vi "KH_DAQ_ReadAll.vi"(8 "err in":errorcluster caption="error", 9 "Debug_DI":bool[](array[boolean]), 10 "Debug_AI":sgl[](array[numeric]), 11 "EIP_AI":T1 {"Offset" format="%.4f"; "Phys Max" format="%.4f"; "Phys Min" format="%.4f"}) -> (0 "err out":errorcluster caption="error")   [LabVIEW 2021]
uses:
  KH_DAQ_TypeDefs_Cluster AI.ctl
  KH_DAQ_TypeDefs_Messbereich.ctl
  KH EthernetIPConfig 17.14/KH EthernetIPConfig TypeDefs ModuleTyp.ctl
  KH_DAQ_TypeDefs_Bereich.ctl
  KH Turck EthernetIP 17.12/KH TURCK TypeDefs FGlob.ctl
  KH EthernetIP 17.19/KH_EthernetIP_Globals.vi
  Turck/KH_DAQ_TURCK_Global.vi
  KH Turck EthernetIP 17.12/KH TURCK ETHERNETIP Global.vi
  KH Turck EthernetIP 17.12/KH TURCK ETHERNETIP RFID Global.vi
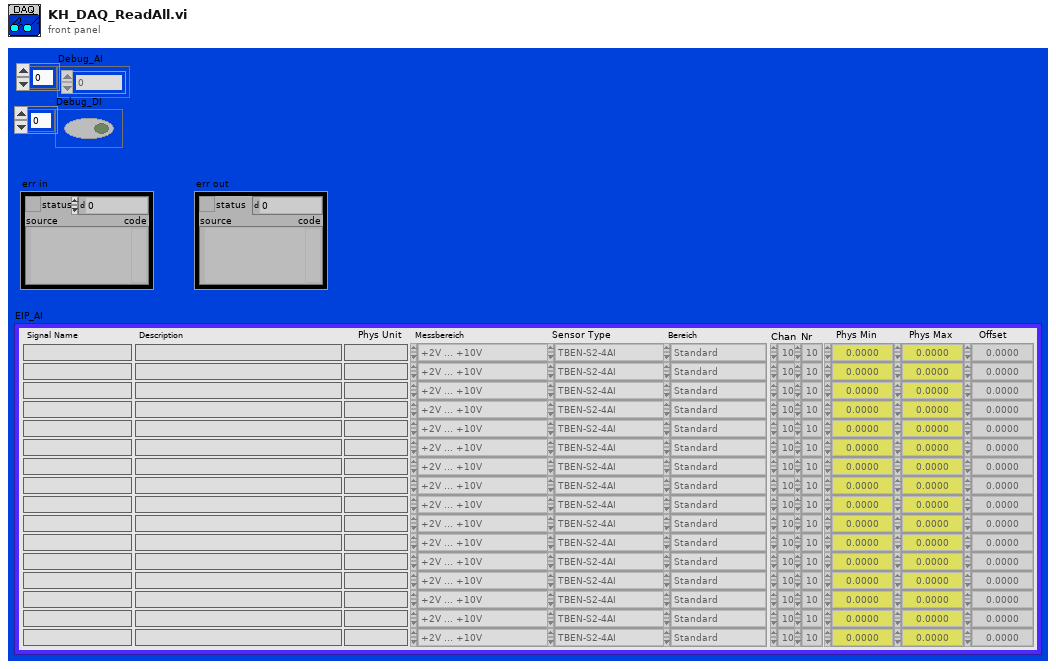
[diagram p1: front panel]
types:
  T1 = typedef "KH_DAQ_TypeDefs_Cluster AI.ctl" = cluster{"Signal Name":string[], "Description":string[], "Phys Unit":string[], "Messbereich":T2[], "Chan":u16[], "Phys Min":sgl[], "Phys Max":sgl[], "Offset":sgl[], "Nr":u16[], "SensorType 2":T3[], "Bereich":T4[]}
  T2 = typedef "KH_DAQ_TypeDefs_Messbereich.ctl" = enum16{"-10V ... +10V", "0V ... +10V", "+2V ... +10V", "0V ... +5V", "+1V ... +5V", "-1V ... +1V", "-500mV ... +500mV", "-100mV ... +100mV", "-50mV ... +50mV", "0mA ... +20mA", "+4mA ... +20mA", "-20mA ... +20mA", "0 Ohm ... 100 Ohm", "0 Ohm ... 400 Ohm", "0 Ohm ... 2000 Ohm", "0 Ohm ... 4000 Ohm", "-200°C ... 150°C PT100", "-200°C ... 150°C PT200", "-200°C ... 150°C PT500", "-200°C ... 150°C PT1000", "-60°C ... 150°C Ni100", "-60°C ... 150°C Ni1000", "-200°C ... 850°C PT100", "-200°C ... 850°C PT200", "-200°C ... 850°C PT500", "-200°C ... 850°C PT1000", "-50°C ... 250°C Ni100", "-50°C ... 250° Ni 1000"}
  T3 = typedef "KH EthernetIPConfig TypeDefs ModuleTyp.ctl" = enum16{"TBEN-S2-4AI", "TBEN-S1-8DXP", "TBEN-S2-2RFID-4DXP", "TBEN-S2-4AO", "TBEN-S2-4IOL"}
  T4 = typedef "KH_DAQ_TypeDefs_Bereich.ctl" = enum16{"Standard", "extended Range", "NE43", ""}
  T5 = typedef "KH TURCK TypeDefs FGlob.ctl" = enum16{"Put one", "Put all", "Recall one", "Recall all"}
  T6 = cluster{"ItemCount":u16, "AdressItem":cluster{"TypeID":u16, "Length":u16, "Data":cluster{"ConnectionIdentifier":u32, "SequenceNumber":u32}}, "DataItem":cluster{"TypeID":u16, "Length":u16, "Data":u8[], "Sequence Count":u16}}
  T7 = typedef "KH EthernetIPConfig TDef Config.ctl" = cluster{"Typ":T3, "Name":string, "Nr.":i32, "InputOutput":enum16{"Input", "Output"}[]}
  T8 = typedef "KH TURCK ETHERNETIP TDefCluster TBEN-S2-4AI Input Values.ctl" = cluster{"Data":i16[], "upper Limit CH0":bool, "upper Limit CH1":bool, "upper Limit CH2":bool, "upper Limit CH3":bool, "Overflow CH0":bool, "Overflow CH1":bool, "Overflow CH2":bool, "Overflow CH3":bool, "Underflow CH0":bool, "Underflow CH1":bool, "Underflow CH2":bool, "Underflow CH3":bool, "CJC Wire Break CH0":bool, "CJC Wire Break CH1":bool, "CJC Wire Break CH2":bool, "CJC Wire Break CH3":bool, "Overcurrent (RTD) CH0":bool, "Overcurrent (RTD) CH1":bool, "Overcurrent (RTD) CH2":bool, "Overcurrent (RTD) CH3":bool, "Wire Break CH0":bool, "Wire Break CH1":bool, "Wire Break CH2":bool, "Wire Break CH3":bool, "Overcurrent supply VAUX1 CH0":bool, "Overcurrent supply VAUX1 CH1":bool, "Overcurrent supply VAUX1 CH2":bool, "Overcurrent supply VAUX1 CH3":bool, "Lower limit value underrun CH0":bool, "Lower limit value underrun CH1":bool, "Lower limit value underrun CH2":bool, "Lower limit value underrun CH3":bool, "Module Diagnostics Available":bool, "INFO: ARGEE Project Running":bool, "Undervoltage Field Supply V2":bool, "Undervoltage Field Supply V1":bool, "Internal Error":bool, "Force Mode Enabled":bool}
  T9 = typedef "KH TURCK ETHERNETIP TDefCluster TBEN-S2-4AO Input Values.ctl" = cluster{"Overload Ch0":bool, "Overload Ch1":bool, "Overload Ch2":bool, "Overload Ch3":bool, "Wirebreak Ch0":bool, "Wirebreak Ch1":bool, "Wirebreak Ch2":bool, "Wirebreak Ch3":bool, "Module Diagnostics Available":bool, "INFO: ARGEE Project Running":bool, "Undervoltage V2":bool, "Undervoltage V1":bool, "Internal Error":bool, "Force Mode Enabled":bool}
  T10 = typedef "KH TURCK ETHERNETIP TDefCluster TBEN-S1-8DXP Input Values.ctl" = cluster{"Data":bool[], "Overcurrent":bool[], "Overcurrent VAUX1 Ch0-3":bool, "Overcurrent VAUX2 Ch4-7":bool, "Latch Input":bool[], "Counter value":u32, "Counter frequency (Hz)":u16, "Status":u8, "Overcurrent PWM Output 3":u8, "Overcurrent PWM Output 7":u8, "Module Diagnostics Available":bool, "INFO: ARGEE Project Running":bool, "Undervoltage V2":bool, "Undervoltage V1":bool, "Force Mode Enabled":bool}
  T11 = typedef "KH TURCK ETHERNETIP TDefCluster TBEN-S2-2RFID-4DXP Input Values.ctl" = cluster{"Station Status Word (Input Data Mapping)":cluster{"Module diagnostics avaliable":bool, "INFO: ARGEE Project Running":bool, "Undervoltage V2":bool, "Undervoltage V1":bool, "Internal Error":bool, "I/O-ASSISTANT Force Mode active":bool}, "RFID control/status 0 (Input Data Mapping)":cluster{"Tag present at r/w head":bool[], "response code":u16, "loop counter":u8, "Length":u16, "Error code":u16, "Tag counter":u16, "Data (Bytes) available":u16, "Read fragment No.":u8, "Write fragment No.":u8, "Tag present at r/w head bit":bool, "HF r/w head switched on":bool, "Continuous mode active":bool, "Antenna detuned at HF read/write head":bool, "Parameter not supported by read/write head":bool, "Error reported by read/write head":bool, "Not connected to read/write head":bool}, "RFID read data 0 (Input Data Mapping)":u8[], "RFID control/status 1 (Input Data Mapping)":cluster{"response code":u16, "Loop counter":u8, "Length":u16, "Error code":u16, "Tag counter":u16, "Data (Bytes) available":u16, "Read fragment No.":u8, "Write fragment No.":u8, "Tag present at r/w head bit":bool, "HF r/w head switched on":bool, "Continuous mode active":bool, "Antenna detuned at HF read/write head":bool, "Parameter not supported by read/write head":bool, "Error reported by read/write head":bool, "Not connected to read/write head":bool, "Tag present at r/w head":bool[]}, "RFID read data 1 (Input Data Mapping)":u8[], "RFID diagnostics (Input Data Mapping)":cluster{"Overcurrent supply VAUX1 (a)":bool, "Parameterization error (a)":bool, "Configuration via DTM active (a)":bool, "Buffer full (a)":bool, "Antenna detuned at HF read/write head (a)":bool[], "Parameter not supported by read/write head (a)":bool[], "Error reported by read/write head (a)":bool[], "Not connected to read/write head (a)":bool[], "Overcurrent supply VAUX1 (b)":bool, "Parameterization error (b)":bool, "Configuration via DTM active (b)":bool, "Buffer full (b)":bool, "Antenna detuned at HF read/write head (b)":bool[], "Parameter not supported by read/write head (b)":bool[], "Error reported by read/write head (b)":bool[], "Not connected to read/write head (b)":bool[]}, "DXP diagnostics (Input Data Mapping)":cluster{"Overcurrent VAUX2 Ch4/5":bool, "Overcurrent VAUX2 Ch6/7":bool, "Channel 4 - Output overcurrent":bool, "Channel 5 - Output overcurrent":bool, "Channel 6 - Output overcurrent":bool, "Channel 7 - Output overcurrent":bool}, "DXP (Input Data Mapping)":cluster{"Channel 4 - Input value":bool, "Channel 5 - Input value":bool, "Channel 6 - Input value":bool, "Channel 7 - Input value":bool}}
  T12 = typedef "KH TURCK ETHERNETIP TDef Enum IOL Data.ctl" = cluster{"Data_Port1":u16[], "Data_Port3":u16[], "Data_Port5":u16[], "Data_Port7":u16[], "Status":cluster{"Undervoltage Field Supply V2":bool, "Overvoltage Field Supply V1":bool, "Undervoltage Field Supply V1":bool, "Internal Error":bool, "Module Diagnostics Available":bool, "Station Configuration Changed":bool, "Overcurrent Isys":bool, "Overvoltage Field Supply V2":bool, "Force Mode Enabled":bool}, "Diagnostics":cluster{"Channel 2 - Output signal overcurrent":bool, "Channel 4 - Output signal overcurrent":bool, "Channel 6 - Output signal overcurrent":bool, "Channel 8 - Output signal overcurrent":bool, "Channel 1 - Wrong or missing device":bool, "Channel 3 - Wrong or missing device":bool, "Channel 5 - Wrong or missing device":bool, "Channel 7 - Wrong or missing device":bool, "Channel 1 - Data storage error":bool, "Channel 3 - Data storage error":bool, "Channel 5 - Data storage error":bool, "Channel 7 - Data storage error":bool, "Channel 1 - Process input data invalid":bool, "Channel 3 - Process input data invalid":bool, "Channel 5 - Process input data invalid":bool, "Channel 7 - Process input data invalid":bool, "Channel 1 - Hardware error":bool, "Channel 3 - Hardware error":bool, "Channel 5 - Hardware error":bool, "Channel 7 - Hardware error":bool, "Channel 1 - Maintenance events":bool, "Channel 3 - Maintenance events":bool, "Channel 5 - Maintenance events":bool, "Channel 7 - Maintenance events":bool, "Channel 1 - Out of spec. error":bool, "Channel 3 - Out of spec. error":bool, "Channel 5 - Out of spec. error":bool, "Channel 7 - Out of spec. error":bool, "Channel 1 - Parameterization error":bool, "Channel 3 - Parameterization error":bool, "Channel 5 - Parameterization error":bool, "Channel 1 - Overtemperature":bool, "Channel 3 - Overtemperature":bool, "Channel 5 - Overtemperature":bool, "Channel 7 - Overtemperature":bool, "Channel 1 - Lower limit value underrun":bool, "Channel 3 - Lower limit value underrun":bool, "Channel 5 - Lower limit value underrun":bool, "Channel 7 - Lower limit value underrun":bool, "Channel 1 - Upper limit value exceeded":bool, "Channel 3 - Upper limit value exceeded":bool, "Channel 5 - Upper limit value exceeded":bool, "Channel 7 - Upper limit value exceeded":bool, "Channel 1 - Undervoltage":bool, "Channel 3 - Undervoltage":bool, "Channel 5 - Undervoltage":bool, "Channel 7 - Undervoltage":bool, "Channel 1 - Overvoltage":bool, "Channel 3 - Overvoltage":bool, "Channel 5 - Overvoltage":bool, "Channel 7 - Overvoltage":bool, "Channel 1 - Overload":bool, "Channel 3 - Overload":bool, "Channel 5 - Overload":bool, "Channel 7 - Overload":bool, "Channel 1 - Common error":bool, "Channel 3 - Common error":bool, "Channel 5 - Common error":bool, "Channel 7 - Common error":bool, "Channel 1 - Port parameterization error":bool, "Channel 3 - Port parameterization error":bool, "Channel 5 - Port parameterization error":bool, "Channel 7 - Parameterization error":bool, "Channel 7 - Port parameterization error":bool}, "Events":cluster{"Event":u8[], "Qualifier":u8[], " Event code":u16[]}, "DXP":cluster{"DI Input value 2":bool, "DI Input value 4":bool, "DI Input value 6":bool, "DI Input value 8":bool, "DI Input 1":bool, "DI Input 3":bool, "DI Input 5":bool, "DI Input 7":bool, "Input values valid 1":bool, "Input values valid 3":bool, "Input values valid 5":bool, "Input values valid 7":bool}}
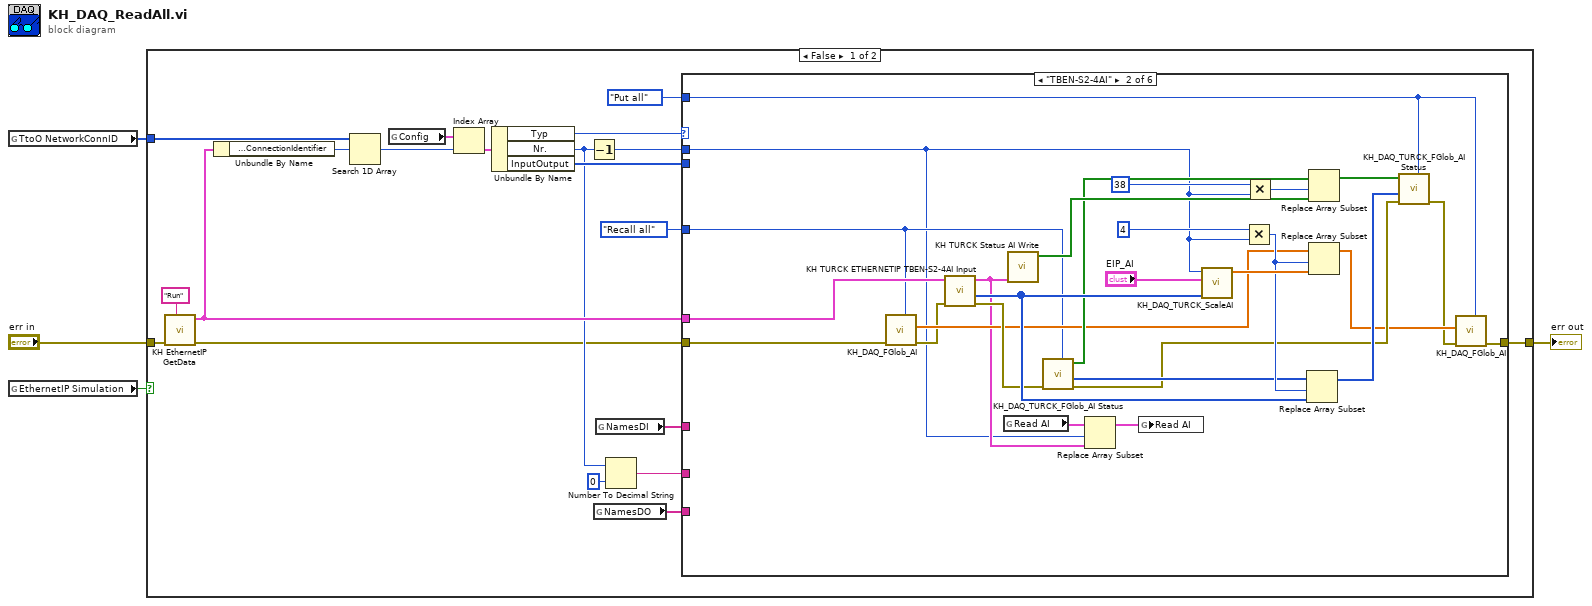
[diagram p0: block diagram]
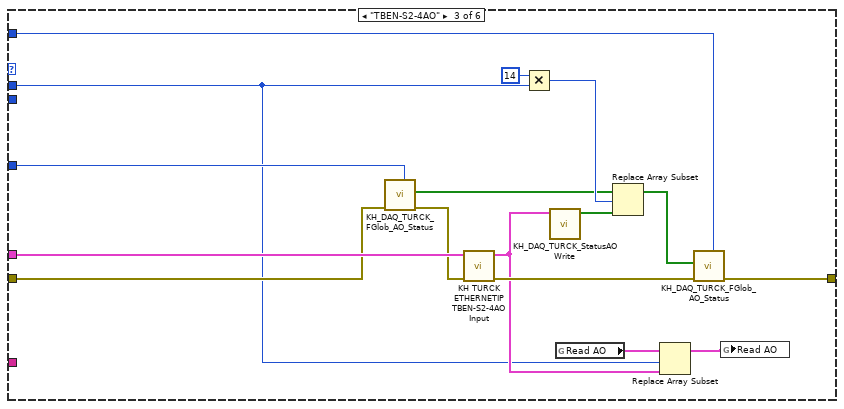
[diagram p3: hidden frame]
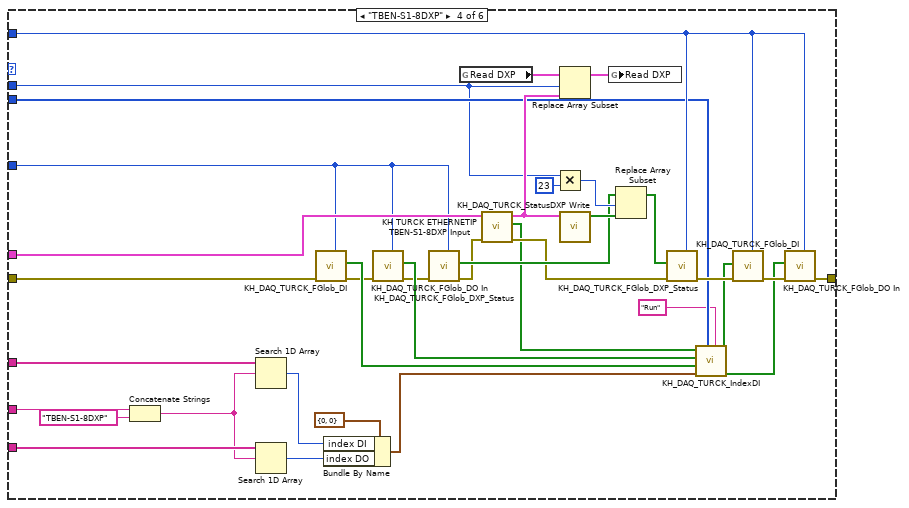
[diagram p4: hidden frame]
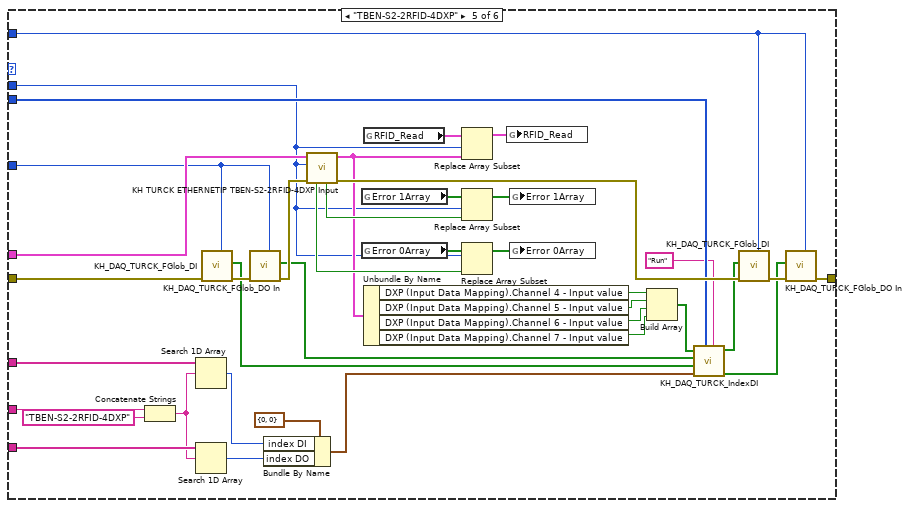
[diagram p5: hidden frame]
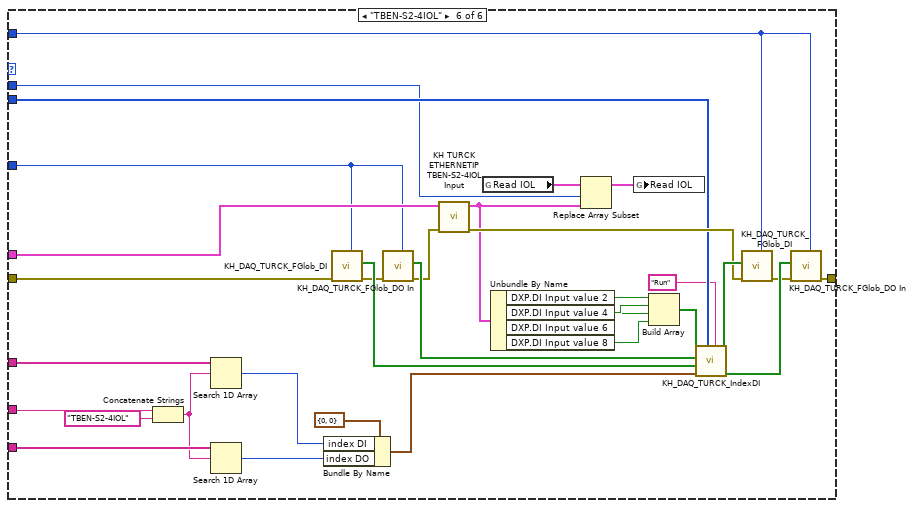
[diagram p6: hidden frame]
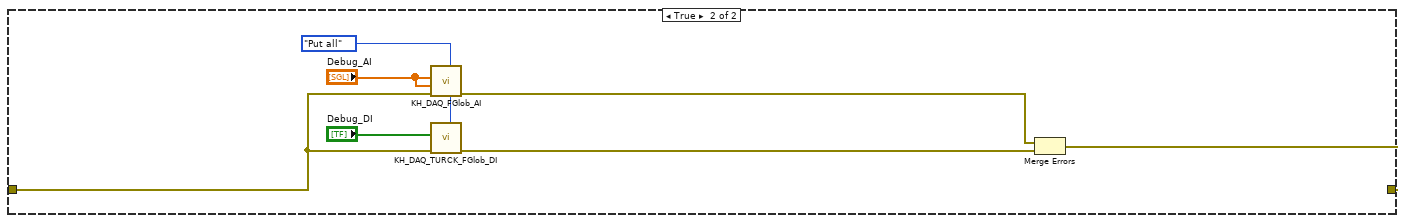
[diagram p7: hidden frame]
diagram:
  n1 = global read "KH_EthernetIP_Globals.vi" "TtoO NetworkConnID"() -> (w2:u32[])
  n2 = global read "KH_EthernetIP_Globals.vi" "EthernetIP Simulation"() -> (w1:bool)
  n3 = case shown="False" w1 {
    tunnel: "err in" -> [w21 w180]
    tunnel: w2 -> [w23 _]
    tunnel: [w13 w179] -> w3
    frame False {
      n4 = call "KH EthernetIP GetData.vi"("Function"="Run", "error in"=w21) -> ("error out"=w6:errorcluster, "Response Data"=w22:T6)  [unwired: 8 in]
      n5 = Unbundle By Name(w22) -> ("AdressItem.Data.ConnectionIdentifier"=w8:u32)
      n6 = Search 1D Array(1D array=w23, element=w8) -> (index of element=w7:i32)  [unwired: 1 in]
      n7 = global read "KH_EthernetIP_Globals.vi" "Config"() -> (w20:T7[])
      n8 = Index Array(array=w20, index=w7) -> (element=w19:T7)
      n9 = Unbundle By Name(w19) -> ("Typ"=w17:T3, "Nr."=w11:i32, "InputOutput"=w16:enum16{"Input", "Output"}[])
      n10 = Decrement(x=w11) -> (x-1=w18:i32)
      n11 = global read "KH_DAQ_TURCK_Global.vi" "NamesDO"() -> (w5:string[])
      n12 = global read "KH_DAQ_TURCK_Global.vi" "NamesDI"() -> (w9:string[])
      n13 = Number To Decimal String(number=w11, width (-)=u16 0 ("Y-Offset")) -> (decimal integer string=w10:string)
      n14 = case shown="\"TBEN-S2-4AI\"" w17 {
        tunnel: w22 -> [_ w52 w68 w104 w137 w176]
        tunnel: w6 -> [w25 w33 w62 w80 w132 w166]
        tunnel: [w25 w36 w57 w92 w128 w163] -> w13
        tunnel: w18 -> [_ w28 w55 w78 w114 w155]
        tunnel: w16 -> [_ _ _ w87 w115 w156]
        tunnel: KH_TURCK_TypeDefs_FGlob."Recall all" ("Function (Recall One)") -> [_ w31 w63 w91 w127 w154]
        tunnel: KH_TURCK_TypeDefs_FGlob."Put all" ("Function (Recall One)") -> [_ w35 w60 w96 w126 w153]
        tunnel: w10 -> [_ _ _ w90 w136 w174]
        tunnel: w9 -> [_ _ _ w88 w134 w173]
        tunnel: w5 -> [_ _ _ w72 w110 w147]
        frame Default {
        }
        frame "TBEN-S2-4AI" {
          n15 = call "KH_DAQ_FGlob_AI.vi"("Function (Recall One)"=w31, "err in"=w33) -> ("err out"=w32:errorcluster, "AI Values OUT"=w34:sgl[])  [unwired: 6 in, 2 out]
          n16 = call "KH TURCK ETHERNETIP TBEN-S2-4AI Input.vi"("error in"=w32, "Response Data"=w52) -> ("error out"=w42:errorcluster, "DataAI"=w49:i16[], "TBEN-S2-4AI Input Values"=w30:T8)  [unwired: 7 in]
          n17 = global read "KH TURCK ETHERNETIP Global.vi" "Read AI"() -> (w26:T8[])
          n18 = call "KH TURCK Status AI Write.vi"("TBEN-S2-4AI Input Values"=w30) -> ("Status"=w48:bool[])  [unwired: 10 in]
          n19 = call "KH_DAQ_TURCK_FGlob_AI Status.vi"("Function (Recall One)"=w31, "err in"=w42) -> ("err out"=w39:errorcluster, "AI Values out unscaled"=w44:i16[], "StatusOut"=w43:bool[])  [unwired: 7 in]
          n20 = Replace Array Subset(array=w26, new element=w30, index=w28) -> (w27:T8[])
          n21 = global write "KH TURCK ETHERNETIP Global.vi" "Read AI"(w27) -> ()
          n22 = call "KH_DAQ_TURCK_ScaleAI.vi"("Messwert Turck"=w49, "EIP_AI"="EIP_AI", "Nr."=w28) -> ("Messwert skaliert"=w51:sgl[])  [unwired: 8 in]
          n23 = Multiply(x=4, y=w28) -> (x*y=w47:i32)
          n24 = Multiply(x=38, y=w28) -> (x*y=w45:i32)
          n25 = Replace Array Subset(array=w44, new element=w49, index=w47) -> (w40:i16[])
          n26 = Replace Array Subset(array=w43, new element=w48, index=w45) -> (w41:bool[])
          n27 = Replace Array Subset(array=w34, new element=w51, index=w47) -> (w38:sgl[])
          n28 = call "KH_DAQ_TURCK_FGlob_AI Status.vi"("Function (Recall One)"=w35, "err in"=w39, "AI Unscaled IN"=w40, "StatusIn"=w41) -> ("err out"=w37:errorcluster)  [unwired: 5 in, 2 out]
          n29 = call "KH_DAQ_FGlob_AI.vi"("Function (Recall One)"=w35, "err in"=w37, "AI Values IN"=w38) -> ("err out"=w36:errorcluster)  [unwired: 5 in, 3 out]
        }
        frame "TBEN-S2-4AO" {
          n30 = call "KH_DAQ_TURCK_FGlob_AO_Status.vi"("Function (Recall One)"=w63, "err in"=w62) -> ("err out"=w61:errorcluster, "AO Status OUT"=w64:bool[])  [unwired: 8 in]
          n31 = call "KH TURCK ETHERNETIP TBEN-S2-4AO Input.vi"("error in"=w61, "Response Data"=w68) -> ("error out"=w58:errorcluster, "TBEN-S2-4AO Input Values"=w56:T9)  [unwired: 8 in]
          n32 = Multiply(x=14, y=w55) -> (x*y=w65:i32)
          n33 = call "KH_DAQ_TURCK_StatusAO Write.vi"("TBEN-S2-4AO Input Values"=w56) -> ("Stauts AO"=w66:bool[])  [unwired: 10 in]
          n34 = global read "KH TURCK ETHERNETIP Global.vi" "Read AO"() -> (w54:T9[])
          n35 = Replace Array Subset(array=w64, new element=w66, index=w65) -> (w59:bool[])
          n36 = Replace Array Subset(array=w54, new element=w56, index=w55) -> (w53:T9[])
          n37 = call "KH_DAQ_TURCK_FGlob_AO_Status.vi"("Function (Recall One)"=w60, "err in"=w58, "AO Status IN"=w59) -> ("err out"=w57:errorcluster)  [unwired: 7 in, 1 out]
          n38 = global write "KH TURCK ETHERNETIP Global.vi" "Read AO"(w53) -> ()
        }
        frame "TBEN-S1-8DXP" {
          n39 = Concatenate Strings(w90, "TBEN-S1-8DXP") -> (w71:string)
          n40 = Search 1D Array(1D array=w88, element=w71) -> (index of element=w70:i32)  [unwired: 1 in]
          n41 = Search 1D Array(1D array=w72, element=w71) -> (index of element=w74:i32)  [unwired: 1 in]
          n42 = call "KH_DAQ_TURCK_FGlob_DI.vi"("Function (Recall One)"=w91, "err in"=w80) -> ("err out"=w81:errorcluster, "DI Values OUT"=w85:bool[])  [unwired: 7 in, 1 out]
          n43 = Bundle By Name(cluster=cluster{"index DI":i32, "index DO":i32} {"index DI"=0, "index DO"=0} ("Index DI DO"), "index DI"=w70, "index DO"=w74) -> (w69:cluster{"index DI":i32, "index DO":i32})
          n44 = call "KH_DAQ_TURCK_FGlob_DO In.vi"("Function (Recall One)"=w91, "err in"=w81) -> ("err out"=w82:errorcluster, "DO in Values OUT"=w86:bool[])  [unwired: 7 in, 1 out]
          n45 = call "KH_DAQ_TURCK_FGlob_DXP_Status.vi"("Function (Recall One)"=w91, "err in"=w82) -> ("err out"=w99:errorcluster, "DXP Status OUT"=w100:bool[])  [unwired: 8 in]
          n46 = global read "KH TURCK ETHERNETIP Global.vi" "Read DXP"() -> (w75:T10[])
          n47 = call "KH TURCK ETHERNETIP TBEN-S1-8DXP Input.vi"("error in"=w99, "Response Data"=w104) -> ("error out"=w97:errorcluster, "DataDXP"=w79:bool[], "TBEN-S1-8DXP Input Values"=w95:T10)  [unwired: 7 in]
          n48 = Multiply(x=w78, y=23) -> (x*y=w101:i32)
          n49 = Replace Array Subset(array=w75, new element=w95, index=w78) -> (w76:T10[])
          n50 = call "KH_DAQ_TURCK_StatusDXP Write.vi"("TBEN-S1-8DXP Input Values"=w95) -> ("Status DXP"=w103:bool[])  [unwired: 10 in]
          n51 = global write "KH TURCK ETHERNETIP Global.vi" "Read DXP"(w76) -> ()
          n52 = Replace Array Subset(array=w100, new element=w103, index=w101) -> (w98:bool[])
          n53 = call "KH_DAQ_TURCK_FGlob_DXP_Status.vi"("Function (Recall One)"=w96, "err in"=w97, "DXP Status IN"=w98) -> ("err out"=w94:errorcluster)  [unwired: 7 in, 1 out]
          n54 = call "KH_DAQ_TURCK_IndexDI.vi"("Function"="Run", "InputOutput"=w87, "Index DI DO"=w69, "DI in"=w85, "DO in in"=w86, "DI Turck"=w79) -> ("DO in out"=w83:bool[], "DI out"=w84:bool[])  [unwired: 4 in]
          n55 = call "KH_DAQ_TURCK_FGlob_DI.vi"("Function (Recall One)"=w96, "err in"=w94, "DI Values IN"=w84) -> ("err out"=w93:errorcluster)  [unwired: 6 in, 2 out]
          n56 = call "KH_DAQ_TURCK_FGlob_DO In.vi"("Function (Recall One)"=w96, "err in"=w93, "DO in Values IN"=w83) -> ("err out"=w92:errorcluster)  [unwired: 6 in, 2 out]
        }
        frame "TBEN-S2-2RFID-4DXP" {
          n57 = Concatenate Strings(w136, "TBEN-S2-2RFID-4DXP") -> (w109:string)
          n58 = Search 1D Array(1D array=w134, element=w109) -> (index of element=w107:i32)  [unwired: 1 in]
          n59 = Search 1D Array(1D array=w110, element=w109) -> (index of element=w106:i32)  [unwired: 1 in]
          n60 = call "KH_DAQ_TURCK_FGlob_DI.vi"("Function (Recall One)"=w127, "err in"=w132) -> ("err out"=w133:errorcluster, "DI Values OUT"=w122:bool[])  [unwired: 7 in, 1 out]
          n61 = call "KH_DAQ_TURCK_FGlob_DO In.vi"("Function (Recall One)"=w127, "err in"=w133) -> ("err out"=w131:errorcluster, "DO in Values OUT"=w123:bool[])  [unwired: 7 in, 1 out]
          n62 = Bundle By Name(cluster=cluster{"index DI":i32, "index DO":i32} {"index DI"=0, "index DO"=0} ("Index DI DO"), "index DI"=w107, "index DO"=w106) -> (w105:cluster{"index DI":i32, "index DO":i32})
          n63 = call "KH TURCK ETHERNETIP TBEN-S2-2RFID-4DXP Input.vi"("error in"=w131, "Nr Modul"=w114, "Response Data"=w137) -> ("error out"=w129:errorcluster, "Cluster"=w121:T11, "Error1"=w143:bool, "Error0"=w138:bool)  [unwired: 2 in, 3 out]
          n64 = global read "KH TURCK ETHERNETIP RFID Global.vi" "Error 1Array"() -> (w142:bool[])
          n65 = global read "KH TURCK ETHERNETIP RFID Global.vi" "Error 0Array"() -> (w139:bool[])
          n66 = global read "KH TURCK ETHERNETIP Global.vi" "RFID_Read"() -> (w112:T11[])
          n67 = Unbundle By Name(w121) -> ("DXP (Input Data Mapping).Channel 4 - Input value"=w120:bool, "DXP (Input Data Mapping).Channel 5 - Input value"=w119:bool, "DXP (Input Data Mapping).Channel 6 - Input value"=w118:bool, "DXP (Input Data Mapping).Channel 7 - Input value"=w117:bool)
          n68 = Replace Array Subset(array=w112, new element=w121, index=w114) -> (w111:T11[])
          n69 = Replace Array Subset(array=w142, new element=w143, index=w114) -> (w141:bool[])
          n70 = Replace Array Subset(array=w139, new element=w138, index=w114) -> (w140:bool[])
          n71 = global write "KH TURCK ETHERNETIP Global.vi" "RFID_Read"(w111) -> ()
          n72 = global write "KH TURCK ETHERNETIP RFID Global.vi" "Error 1Array"(w141) -> ()
          n73 = global write "KH TURCK ETHERNETIP RFID Global.vi" "Error 0Array"(w140) -> ()
          n74 = Build Array(w120, w119, w118, w117) -> (w116:bool[])
          n75 = call "KH_DAQ_TURCK_IndexDI.vi"("Function"="Run", "InputOutput"=w115, "Index DI DO"=w105, "DI in"=w122, "DO in in"=w123, "DI Turck"=w116) -> ("DO in out"=w124:bool[], "DI out"=w125:bool[])  [unwired: 4 in]
          n76 = call "KH_DAQ_TURCK_FGlob_DI.vi"("Function (Recall One)"=w126, "err in"=w129, "DI Values IN"=w125) -> ("err out"=w130:errorcluster)  [unwired: 6 in, 2 out]
          n77 = call "KH_DAQ_TURCK_FGlob_DO In.vi"("Function (Recall One)"=w126, "err in"=w130, "DO in Values IN"=w124) -> ("err out"=w128:errorcluster)  [unwired: 6 in, 2 out]
        }
        frame "TBEN-S2-4IOL" {
          n78 = Concatenate Strings(w174, "TBEN-S2-4IOL") -> (w146:string)
          n79 = Search 1D Array(1D array=w173, element=w146) -> (index of element=w145:i32)  [unwired: 1 in]
          n80 = Search 1D Array(1D array=w147, element=w146) -> (index of element=w149:i32)  [unwired: 1 in]
          n81 = Bundle By Name(cluster=cluster{"index DI":i32, "index DO":i32} {"index DI"=0, "index DO"=0} ("Index DI DO"), "index DI"=w145, "index DO"=w149) -> (w144:cluster{"index DI":i32, "index DO":i32})
          n82 = call "KH_DAQ_TURCK_FGlob_DI.vi"("Function (Recall One)"=w154, "err in"=w166) -> ("err out"=w167:errorcluster, "DI Values OUT"=w172:bool[])  [unwired: 7 in, 1 out]
          n83 = call "KH_DAQ_TURCK_FGlob_DO In.vi"("Function (Recall One)"=w154, "err in"=w167) -> ("err out"=w165:errorcluster, "DO in Values OUT"=w171:bool[])  [unwired: 7 in, 1 out]
          n84 = call "KH TURCK ETHERNETIP TBEN-S2-4IOL Input.vi"("error in"=w165, "Response Data"=w176) -> ("error out"=w164:errorcluster, "Data_IOL"=w162:T12)  [unwired: 8 in]
          n85 = global read "KH TURCK ETHERNETIP Global.vi" "Read IOL"() -> (w150:T12[])
          n86 = Unbundle By Name(w162) -> ("DXP.DI Input value 2"=w161:bool, "DXP.DI Input value 4"=w160:bool, "DXP.DI Input value 6"=w159:bool, "DXP.DI Input value 8"=w158:bool)
          n87 = Replace Array Subset(array=w150, new element=w162, index=w155) -> (w151:T12[])
          n88 = global write "KH TURCK ETHERNETIP Global.vi" "Read IOL"(w151) -> ()
          n89 = Build Array(w161, w160, w159, w158) -> (w157:bool[])
          n90 = call "KH_DAQ_TURCK_IndexDI.vi"("Function"="Run", "InputOutput"=w156, "Index DI DO"=w144, "DI in"=w172, "DO in in"=w171, "DI Turck"=w157) -> ("DO in out"=w170:bool[], "DI out"=w169:bool[])  [unwired: 4 in]
          n91 = call "KH_DAQ_TURCK_FGlob_DI.vi"("Function (Recall One)"=w153, "err in"=w164, "DI Values IN"=w169) -> ("err out"=w168:errorcluster)  [unwired: 6 in, 2 out]
          n92 = call "KH_DAQ_TURCK_FGlob_DO In.vi"("Function (Recall One)"=w153, "err in"=w168, "DO in Values IN"=w170) -> ("err out"=w163:errorcluster)  [unwired: 6 in, 2 out]
        }
      }
    }
    frame True {
      w181 = KH_TURCK_TypeDefs_FGlob."Put all" ("Function (Recall One)")
      n93 = call "KH_DAQ_FGlob_AI.vi"("Function (Recall One)"=w181, "err in"=w180, "AI Unscaled IN"="Debug_AI", "AI Values IN"="Debug_AI") -> ("err out"=w182:errorcluster)  [unwired: 4 in, 3 out]
      n94 = call "KH_DAQ_TURCK_FGlob_DI.vi"("Function (Recall One)"=w181, "err in"=w180, "DI Values IN"="Debug_DI") -> ("err out"=w183:errorcluster)  [unwired: 6 in, 2 out]
      n95 = Merge Errors(w182, w183) -> (w179:errorcluster)
    }
  }
  "err out" <- w3
